vi "Initial Condition.vi"   [LabVIEW 2020, in "NI_AdvCtrl_nonlinear.lvlib"]
doc: "LabVIEW no longer supports this VI. You can obtain similar functionality by installing the LabVIEW Simulation Module.\n\nProduces a predefined initial condition immediately after the first call."
uses:
  <vilib>/addons/control/advanced/NI_AdvCtrl_nonlinear.lvlib
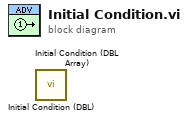
[diagram p0: block diagram]
diagram:
  n1 = call <vilib>:"Initial Condition (DBL).vi"() -> ()  [unwired: 5 in, 1 out]
  n2 = call <vilib>:"Initial Condition (DBL Array).vi"() -> ()  [unwired: 5 in, 1 out]
